vi "LIA with AM10.vi"() -> ()   [LabVIEW 2013]
uses:
  <vilib>/express/express analysis/Spectral/Block/exnSpectralBlock spectral measurements power poly.vi
  <vilib>/express/express analysis/Spectral/Block/exnSpectralBlock spectral measurements power WFM.vi
  <vilib>/express/express analysis/Spectral/XNode/ExpressSpectralMeasurementsBlockNode.xnode
panel:
  out "XY output":dbl[][](graph)=[[7.160796582041422e-23, 0.8613310626146382, 2.4561359846943875, 2.952874741807238, 1.7810719719127623, 0.28647450836648075, 0.1855399799266717, 1.5941857793632301, 2.8946647286877365, 2.5934529411128726, 1.0364745084779694, 0.011827948025126142, 0.696259807484987, 2.3037401923711305, 2.9881720520319566, 1.9635254917181835, 0.406547058891952, 0.1053352711626314, 1.405814220670607, 2.8144600200045553, 2.7135254917289764, 1.2189280280935204, 0.047125258287880584, 0.5438640153388544, 2.138668937250768, 2.999999999813988, 2.138668937326914, 0.5438640153438781, 0.04712525829527701, 1.2189280280673727, 2.7135254915392104, 2.8144600200446352, 1.405814220676119, 0.10533527116920109, 0.4065470588630961, 1.96352549160863, 2.9881720520128687, 2.3037401926017003, 0.6962598075630243, 0.011827948035904793, 1.0364745085201217, 2.593452941203313, 2.8946647287738734, 1.594185779237936, 0.18553997990325743, 0.2864745084519614, 1.7810719718442396, 2.9528747414006133, 2.4561359846600666, 0.861331062670481, 3.3077676520313965e-24, 0.8613310627550416, 2.4561359846139497, 2.9528747415820673, 1.7810719718610435, 0.28647450845342576, 0.18553997990881135, 1.5941857791936822, 2.8946647285307203, 2.5934529411452028, 1.0364745085708484, 0.01182794802446571, 0.6962598076358434, 2.3037401924693217, 2.9881720519815427, 1.9635254914432874, 0.4065470589446706, 0.10533527118504565, 1.4058142206375985, 2.814460020130084, 2.7135254916593086, 1.2189280280503507, 0.04712525828537252, 0.5438640154419273, 2.1386689373343555, 3.0000000000990474, 2.1386689374412686, 0.5438640154158645, 0.04712525831168253, 1.2189280280960597, 2.7135254916498694, 2.814460020186744, 1.4058142207416613, 0.10533527116967795, 0.40654705886722364, 1.963525491642289, 2.988172052072964, 2.3037401923713547, 0.6962598075051848, 0.011827948028521627, 1.036474508509565, 2.593452941035456, 2.894664728876174, 1.5941857792833374, 0.18553997989479157, 0.28647450845309624, 1.7810719719307495, 2.9528747417073142, 2.456135984617047, 0.8613310626750714], [6.397055649297223e-11, 1.3572405786433024, 1.1557698641977745, -0.3730348307598141, -1.4734308761192492, -0.8816778782179262, 0.7226305111206902, 1.4970400927124303, 0.5521868290009423, -1.0268206588885556, -1.4265847744961446, -0.1879998502992948, 1.266491888166919, 1.266491888200227, -0.18799985034798364, -1.4265847745588331, -1.0268206589514395, 0.5521868289985771, 1.4970400926044023, 0.7226305111386365, -0.8816778784900925, -1.4734308760566728, -0.3730348305927203, 1.155769864081423, 1.3572405786439674, 2.6015694700992775e-12, -1.3572405786883703, -1.1557698640905518, 0.37303483065207627, 1.473430876027617, 0.8816778784332103, -0.7226305111440005, -1.497040092612899, -0.5521868290321227, 1.0268206588799003, 1.426584774477441, 0.18799985035196828, -1.2664918883228173, -1.2664918883125516, 0.18799985047137116, 1.4265847745564424, 1.0268206589180475, -0.5521868290123274, -1.4970400925916614, -0.7226305110339414, 0.881677878482172, 1.473430876065951, 0.37303483070812155, -1.1557698641772307, -1.3572405787292774, 7.286958480330694e-12, 1.357240578861082, 1.1557698641619196, -0.3730348307293721, -1.473430876074467, -0.8816778784889762, 0.722630511058582, 1.497040092549754, 0.5521868289675292, -1.0268206588939026, -1.4265847746274427, -0.18799985028680116, 1.266491888443322, 1.2664918882562046, -0.18799985034827246, -1.4265847743516558, -1.0268206590880522, 0.552186829118073, 1.4970400925712481, 0.7226305111728633, -0.8816778784709165, -1.473430876002493, -0.3730348305763276, 1.1557698642970033, 1.3572405786935529, -8.590198202405667e-13, -1.3572405787589454, -1.1557698642469916, 0.3730348307839356, 1.4734308760588328, 0.8816778784711621, -0.7226305111839482, -1.4970400926806984, -0.5521868290380831, 1.0268206588923217, 1.426584774503892, 0.1879998503577455, -1.2664918881996443, -1.2664918881998886, 0.18799985035055852, 1.4265847745384521, 1.0268206588590414, -0.5521868290353029, -1.4970400926322998, -0.7226305109989726, 0.8816778784876612, 1.4734308761340573, 0.37303483075432026, -1.1557698641604481, -1.3572405787345143]] caption="Input Signal"
  out "Lock-in Output":cluster{"Ch 1 Output":dbl, "Ch 2 Output":dbl}(graph)={"Ch 1 Output"=2.99999147666684, "Ch 2 Output"=4.749187889468861e-12} caption="Lock-in Analysis"
  in  "Phase (°)":dbl caption="LOCK-IN Phase" format="%.2f"
  in  "Monitor":u16(ring) items=["Input Signal", "After Mixer"]
  out "Power Spectral Density":cluster{"f0":dbl, "df":dbl, "magnitude":dbl[]}(graph)={"f0"=0.0, "df"=0.01, "magnitude"=[-235.21607825145085, -218.3937535918811, -211.57980464454627, -219.0173516225138, -216.7688290117615, -227.34685181005236, -218.16724192412624, -214.6758364793697, -214.71830862190149, 9.542425094407328, -217.7051009330383, -220.7691633252297, -212.60929639110955, -213.01249803295275, -216.67836056343054, -214.9995950002794, -220.6607411225575, -212.65395812587005, -224.25144059753904, -218.23736966151543, -219.96657196923883, -222.76781056167866, -212.8404028730375, -214.7157786100669, -210.0824382535258, -215.8244598071573, -209.1926052730962, -211.51409381734052, -221.9697489273974, -215.1870579937338, -211.0080371535637, -230.61801872432034, -222.61555635556283, -215.12031239654422, -226.3222143787744, -213.08361230290757, -213.73344693439827, -212.09149744828164, -237.98927548601935, -221.72257852706096, -216.38992841637275, -214.7673342129894, -215.80884880067177, -207.499972356578, -215.86127934217419, -219.33399937224, -219.58911586802202, -216.03742266424695, -215.02006922582063, -218.03690366453156]}
  out "Phasor Representation of Lock-In Output":cluster{"Ch 1 Output":dbl, "Ch 2 Output":dbl}[](graph)=[{"Ch 1 Output"=2.99662702723827, "Ch 2 Output"=-2.5790815749905384e-12}, {"Ch 1 Output"=2.995358935904702, "Ch 2 Output"=-1.600659266616595e-12}, {"Ch 1 Output"=2.9945927518921893, "Ch 2 Output"=-1.1586173268220065e-12}, {"Ch 1 Output"=2.994229007813994, "Ch 2 Output"=-1.0891180515438528e-12}, {"Ch 1 Output"=2.994178400041988, "Ch 2 Output"=-7.018571078375837e-13}, {"Ch 1 Output"=2.9943625860211864, "Ch 2 Output"=1.2387460212332801e-13}, {"Ch 1 Output"=2.9947143595459833, "Ch 2 Output"=9.988247092988941e-13}, {"Ch 1 Output"=2.9951773567757507, "Ch 2 Output"=1.6429471635901913e-12}, {"Ch 1 Output"=2.9957054244850045, "Ch 2 Output"=2.3074000163604176e-12}, {"Ch 1 Output"=2.9962617612040914, "Ch 2 Output"=3.132801941572091e-12}, {"Ch 1 Output"=2.9968179221936446, "Ch 2 Output"=3.8173071586339545e-12}, {"Ch 1 Output"=2.9973527610714332, "Ch 2 Output"=3.922307228194296e-12}, {"Ch 1 Output"=2.9978513646575764, "Ch 2 Output"=3.2926514915426665e-12}, {"Ch 1 Output"=2.998304023363372, "Ch 2 Output"=2.5213873287780478e-12}, {"Ch 1 Output"=2.9987052672430683, "Ch 2 Output"=2.095662338336086e-12}, {"Ch 1 Output"=2.9990529876049297, "Ch 2 Output"=1.7451639948826307e-12}, {"Ch 1 Output"=2.9993476557183225, "Ch 2 Output"=1.0766983637301205e-12}, {"Ch 1 Output"=2.9995916434977667, "Ch 2 Output"=-7.7713426602266e-14}, {"Ch 1 Output"=2.9997886459053773, "Ch 2 Output"=-1.4843901385551484e-12}, {"Ch 1 Output"=2.9999432010043945, "Ch 2 Output"=-2.805711784224486e-12}, {"Ch 1 Output"=3.000060300921067, "Ch 2 Output"=-4.182689754747923e-12}, {"Ch 1 Output"=3.0001450852334033, "Ch 2 Output"=-5.7840254493691e-12}, {"Ch 1 Output"=3.000202607338317, "Ch 2 Output"=-7.433486148990116e-12}, {"Ch 1 Output"=3.0002376639933472, "Ch 2 Output"=-8.674989772490261e-12}, {"Ch 1 Output"=3.000254678334139, "Ch 2 Output"=-9.056488928793801e-12}, {"Ch 1 Output"=3.000257627115586, "Ch 2 Output"=-8.692276282347365e-12}, {"Ch 1 Output"=3.000250003613007, "Ch 2 Output"=-8.104261962935539e-12}, {"Ch 1 Output"=3.0002348084548918, "Ch 2 Output"=-7.494134437440875e-12}, {"Ch 1 Output"=3.0002145615773665, "Ch 2 Output"=-6.9560421124757496e-12}, {"Ch 1 Output"=3.00019132943091, "Ch 2 Output"=-6.736480378543125e-12}, {"Ch 1 Output"=3.0001667624899815, "Ch 2 Output"=-6.884063964721238e-12}, {"Ch 1 Output"=3.000142138997351, "Ch 2 Output"=-7.347238916487514e-12}, {"Ch 1 Output"=3.000118411679514, "Ch 2 Output"=-8.014782704962025e-12}, {"Ch 1 Output"=3.0000962548898635, "Ch 2 Output"=-8.601127070451612e-12}, {"Ch 1 Output"=3.0000761102732425, "Ch 2 Output"=-8.847007531240794e-12}, {"Ch 1 Output"=3.000058229590788, "Ch 2 Output"=-8.936320334688542e-12}, {"Ch 1 Output"=3.000042713802999, "Ch 2 Output"=-8.927590533950898e-12}, {"Ch 1 Output"=3.000029547880391, "Ch 2 Output"=-8.239303128363778e-12}, {"Ch 1 Output"=3.0000186311090906, "Ch 2 Output"=-6.696268700027832e-12}, {"Ch 1 Output"=3.0000098028931537, "Ch 2 Output"=-4.771497592300238e-12}, {"Ch 1 Output"=3.0000028642245966, "Ch 2 Output"=-2.808072656482772e-12}, {"Ch 1 Output"=2.9999975951124305, "Ch 2 Output"=-8.15920048923648e-13}, {"Ch 1 Output"=2.9999937683435385, "Ch 2 Output"=1.160281416825983e-12}, {"Ch 1 Output"=2.9999911599920828, "Ch 2 Output"=2.5866747361203684e-12}, {"Ch 1 Output"=2.9999895571091137, "Ch 2 Output"=3.0453247859602903e-12}, {"Ch 1 Output"=2.999988763022408, "Ch 2 Output"=2.99657373707623e-12}, {"Ch 1 Output"=2.999988600658461, "Ch 2 Output"=3.25905893169565e-12}, {"Ch 1 Output"=2.999988914265522, "Ch 2 Output"=4.051312205799775e-12}, {"Ch 1 Output"=2.999989569881677, "Ch 2 Output"=4.7268767433370936e-12}, {"Ch 1 Output"=2.9999904548535827, "Ch 2 Output"=4.886296431704625e-12}] caption="XY Graph"
  out "Time-Domain":dbl[][](graph)=[[5.7264905182118526e-11, 1.6074803850291068, 2.714481157375272, 2.976344103913628, 2.311539728422606, 0.9270509830904567, -0.7460696614724398, -2.1869058822716396, -2.9468617524061633, -2.789329457711673, -1.7633557568847291, -0.18837155849797071, 1.445261022346591, 2.628920040335509, 2.994080185279943, 2.427050983244081, 1.1043736580146353, -0.5621439439077028, -2.053641317613207, -2.905749483311644, -2.853169548811224, -1.912271969373071, -0.37599970068327676, 1.277337874669322, 2.5329837765284298, 2.999999999929249, 2.532983776596802, 1.2773378747838027, -0.3759997008364309, -1.9122719691652454, -2.85316954893021, -2.9057494834195046, -2.053641317725618, -0.5621439439232003, 1.1043736580337347, 2.427050983043902, 2.994080185337669, 2.6289200401578983, 1.4452610221701134, -0.1883715586287009, -1.7633557568382405, -2.789329457700561, -2.946861752358229, -2.1869058821346656, -0.7460696615691468, 0.9270509830480291, 2.3115397283942496, 2.9763441039140974, 2.714481157331208, 1.6074803848424404, 3.1941014126547703e-12, -1.607480384929976, -2.7144811573655114, -2.9763441038477843, -2.31153972845064, -0.9270509831065624, 0.7460696613477636, 2.1869058823191936, 2.946861752084573, 2.7893294576862684, 1.7633557570309557, 0.1883715587352395, -1.445261022233788, -2.6289200402198905, -2.99408018525837, -2.4270509830062603, -1.1043736580309171, 0.5621439437525994, 2.0536413177121613, 2.905749483546511, 2.853169548964771, 1.9122719691992385, 0.3759997007175391, -1.2773378745019865, -2.532983776459921, -3.000000000086837, -2.5329837766539796, -1.2773378745456503, 0.3759997006264955, 1.9122719691101928, 2.8531695489636224, 2.905749483361673, 2.0536413177483404, 0.5621439437392151, -1.1043736580438444, -2.427050983158539, -2.9940801853415446, -2.628920040177921, -1.4452610222029727, 0.18837155865800395, 1.7633557568570961, 2.7893294575180625, 2.9468617522226395, 2.1869058821760277, 0.7460696614997623, -0.9270509831169068, -2.3115397282190187, -2.976344103874128, -2.714481157489229, -1.6074803848518553], [-2.17504699296209e-13, 0.5358267949785253, 0.9048270524664113, 0.9921147013144053, 0.7705132427756372, 0.3090169943750446, -0.24868988716530674, -0.7289686274214977, -0.9822872507286484, -0.9297764858881211, -0.5877852522924625, -0.06279051952964025, 0.48175367410192665, 0.8763066800438156, 0.9980267284282992, 0.8090169943748718, 0.3681245526848752, -0.18738131458518154, -0.6845471059293632, -0.9685831611287765, -0.9510565162950781, -0.6374239897487644, -0.12533323356383602, 0.4257792915651914, 0.8443279255019028, 1.0, 0.8443279255020052, 0.4257792915653642, -0.12533323356454887, -0.6374239897486171, -0.9510565162950192, -0.9685831611285978, -0.6845471059288395, -0.1873813145862625, 0.3681245526855433, 0.8090169943752942, 0.9980267284282872, 0.8763066800439077, 0.48175367410129705, -0.06279051952944965, -0.5877852522923079, -0.9297764858883856, -0.9822872507286842, -0.7289686274216284, -0.2486898871646108, 0.30901699437486296, 0.7705132427755155, 0.9921147013144953, 0.9048270524661053, 0.5358267949794544, -9.360250641947212e-13, -0.5358267949794993, -0.9048270524661279, -0.9921147013144886, -0.7705132427754816, -0.3090169943748125, 0.2486898871646622, 0.7289686274216648, 0.9822872507286942, 0.929776485888366, 0.587785252292265, 0.0627905195293967, -0.4817536741013435, -0.8763066800439332, -0.9980267284282839, -0.809016994375263, -0.368124552685494, 0.18738131458631463, 0.6845471059288781, 0.968583161128611, 0.9510565162950028, 0.6374239897485763, 0.12533323356449624, -0.42577929156541217, -0.8443279255020336, -1.0, -0.8443279255018744, -0.4257792915651434, 0.12533323356388867, 0.6374239897488052, 0.9510565162950946, 0.9685831611287633, 0.6845471059293246, 0.1873813145851294, -0.36812455268492456, -0.809016994374903, -0.9980267284283025, -0.8763066800437901, -0.4817536741018802, 0.06279051952969321, 0.5877852522925053, 0.9297764858881407, 0.9822872507286384, 0.7289686274214614, 0.24868988716525536, -0.30901699437509506, -0.770513242775671, -0.9921147013144119, -0.9048270524663886, -0.5358267949784805]] caption="Input Signal"
  in  "Tab Control":enum32{"Main Settings ", "Other Settings"}(tab)
  in  "Sinusoidal\nInput\nSettings":cluster{"fc (Hz)":dbl, "Ac (V)":dbl}[](array[cluster])=[{"fc (Hz)"=60.0, "Ac (V)"=1.0}]
  out "CH Y Output (V)":dbl(knob)=4.749187889468861e-12 caption="CH 2 Output" scale=-5.0..5.0
  out "CH X Output (V)":dbl(knob)=2.99999147666684 caption="CH 1 Output" scale=-5.0..5.0
  in  "Frequency fS (Hz)":dbl=90.0 caption="Frequency" format="%.2f"
  in  "Amplitude AS (V)":dbl=3.0 caption="Amplitude" format="%.2f"
  in  "AM Percentage (%)":dbl caption="Noise Amplitude" min=0.0 max=100.0
  in  "Phase  f (°)":dbl caption="Phase Angle" format="%.2f"
  in  "AM Freq fAM (Hz)":dbl=1.0 caption="Noise Amplitude" format="%.4f"
  in  "Auto-Track":bool=TRUE caption="Auto-Tracking"
  in  "Low-Pass Filter":bool=TRUE
  in  "Time Constant t (s)":dbl=3.0 caption="Time Constant (sec)" format="%#.1p"
  in  "Rolloff":sgl(ring)=2.0 caption="Low-pass filter slope" items=["None", "6 dB/oct", "12 dB/oct", "18 dB/oct", "24 dB/oct"]
  in  "Ref  Freq  fR (Hz)":dbl=90.0 caption="Manual Set" format="%.2f"
  in  "(V)":dbl=1e-11 caption="Noise Amplitude" min=1e-11 format="%.4f"
  in  "Enable sinusoidal inputs":bool
  out "Ch 1 Output":dbl=2.99999147666684 format="%.2f"
  out "Ch 2 Output":dbl=4.749187889468861e-12 format="%.2f"
  out "Magnitude":dbl=2.99999147666684 caption="Input Signal Amp" format="%.2f"
  out "Phase":dbl=9.070306509121702e-11 caption="Phase Difference" format="%.2f"
  out "Sampling Freq.":dbl=1000.0 format="%.2f"
  in  "IntegrationPeriod(s)":dbl=0.1 format="%#_6p"
  in  "Sampling Int. (s)":dbl=0.001 caption="Sampling Int. (ms)" format="%.3f"
  # ","
  # "Input Signal"
  # "Lockin Output"
  # "Lockin Settings"
  # "Additional Signals"
  # "noise"
  # "Lock-In Output"
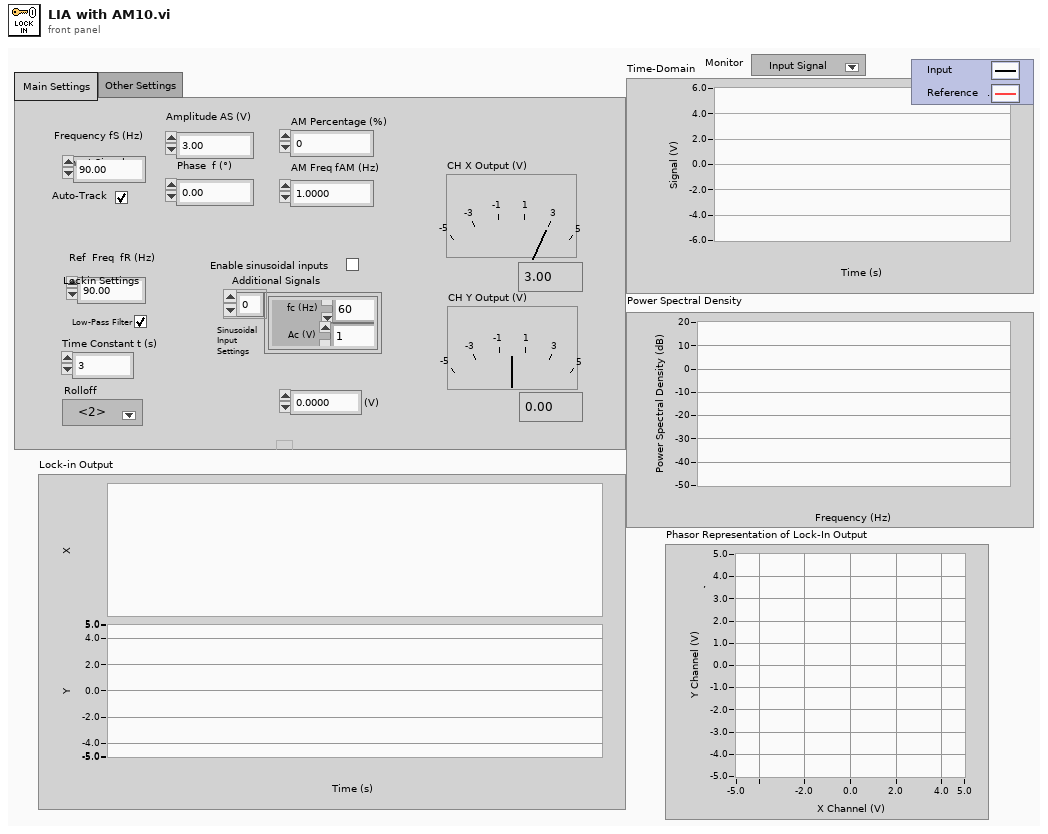
[diagram p1: front panel]
types:
  T1 = cluster{"averaging mode":u16, "weighting mode":u16, "number of averages":u32}
  T2 = cluster{"dB On (F)":bool, "unwrap phase (F)":bool, "convert to degree (F)":bool}
  T3 = cluster{"Amplitude AS (V)":dbl, " Frequency fS (Hz)":dbl, "Phase  f (°)":dbl, dbl, "Rolloff":sgl, "Time Constant t (s)":dbl, bool, " Phase (°)":dbl, " Frequency fS (Hz)":dbl, dbl, "AM Freq fAM (Hz)":dbl, "Sampling Int. (s)":dbl, dbl}
  T4 = cluster{"Amplitude":dbl, "Frequency":dbl, "Phase Angle":dbl, "Spectral Amplitude":dbl, "Time":dbl, "Low-pass filter scope":dbl, "Time Constant (sec)":dbl, "Reset Filters":bool, "LOCK-IN Phase":dbl, "LOCK-IN Freq":dbl, "Sampling-Int(ms)":dbl, "Reference Signal":cluster{dbl[], dbl[]}, "Input Signal":dbl[], "N":i32}
  T5 = cluster{"Amplitude":dbl, "Frequency":dbl, "Phase Angle":dbl, "Noise Amplitude":dbl, "Time":dbl, "Low-pass filter slope":dbl, "Time Constant (sec)":dbl, "Reset Filters":bool, "LOCK-IN Phase":dbl, "LOCK-IN Freq":dbl, "Input Signal":dbl[], "Ch 1 Mult":dbl, "Ch 2 Mult":dbl, "Reference Signal":cluster{dbl[], dbl[]}}
  T6 = cluster{"Ch 1 Output":dbl, "Ch 2 Output":dbl, "Input Signal Amp":dbl, "Phase Difference":dbl, "X-Y Data":cluster{"Current Queue":dbl[], "Current Queue":dbl[]}, "Input Signal":dbl[], "Reference Signal":cluster{dbl[], dbl[]}}
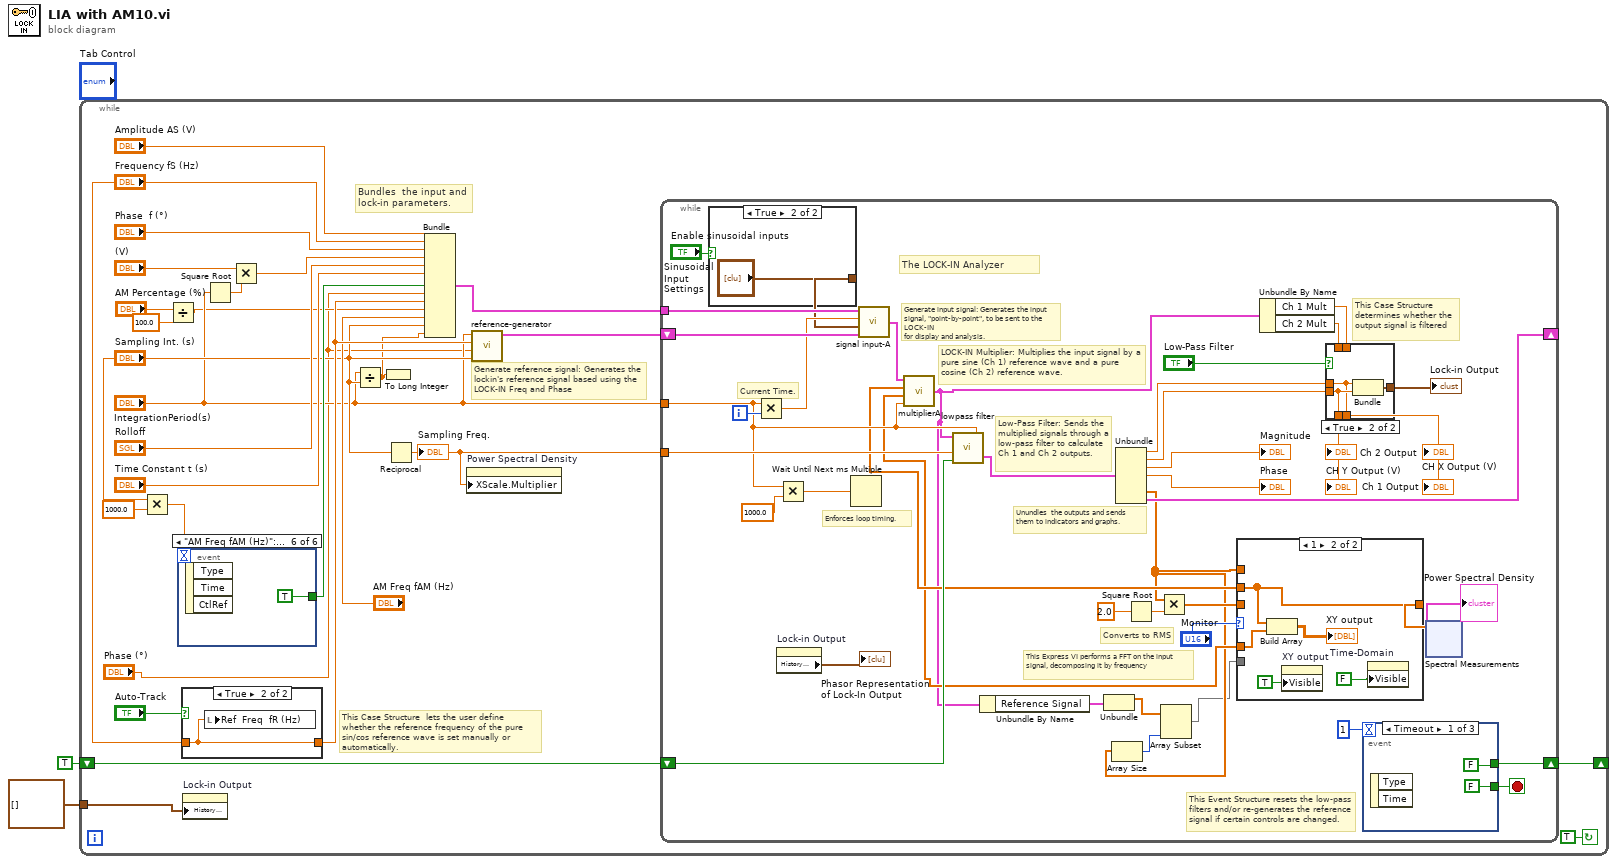
[diagram p0: block diagram]
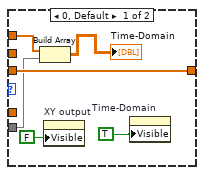
[diagram p2: hidden frame]
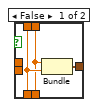
[diagram p3: hidden frame]
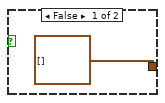
[diagram p4: hidden frame]
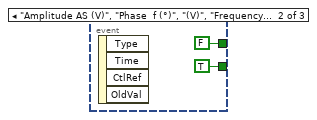
[diagram p5: hidden frame]
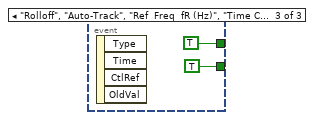
[diagram p6: hidden frame]
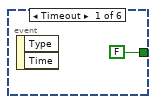
[diagram p7: hidden frame]
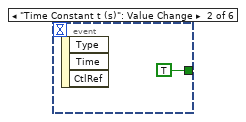
[diagram p8: hidden frame]
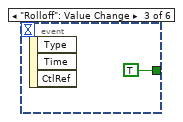
[diagram p9: hidden frame]
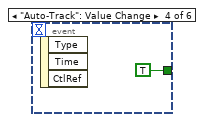
[diagram p10: hidden frame]
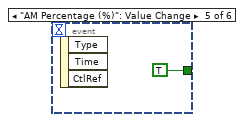
[diagram p11: hidden frame]
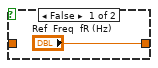
[diagram p12: hidden frame]
diagram:
  n1 = while {
    shift-right: [w22] -> _
    shift-left: TRUE -> [w23]
    tunnel: cluster{"Ch 1 Output":dbl, "Ch 2 Output":dbl}[] [] ("History Data") -> [w4]
    stop <- TRUE continue-if-true
    # "Generate reference signal: Generates the \nlockin's reference signal based using the \nLOCK-IN Freq and Phase"
    # "This Case Structure  lets the user define whether the reference frequency of the pure sin/cos reference wave is set manually or automatically."
    # "Bundles  the input and lock-in parameters."
    n2 = Multiply(x="Sampling Int. (s)", y=1000.0) -> (x*y=w16:dbl)
    n3 = Divide(x="AM Percentage (%)", y=100.0) -> (x/y=w6:dbl)
    n4 = event shown="[5] \"AM Freq fAM (Hz)\": Value Change" {
      selector: _ -> [_ _ _ _ _ _]
      dyn-events: _ -> [_ _ _ _ _ _]
      timeout: w16 -> [_ _ _ _ _ _]
      tunnel: [FALSE TRUE TRUE TRUE TRUE TRUE] -> w19
      event Timeout {
        n5 = event-data() -> ()  [unwired: 1 in, 2 out]
      }
      event "Time Constant t (s)": Value Change {
        n6 = event-data() -> ()  [unwired: 1 in, 3 out]
      }
      event "Rolloff": Value Change {
        n7 = event-data() -> ()  [unwired: 1 in, 3 out]
      }
      event "Auto-Track": Value Change {
        n8 = event-data() -> ()  [unwired: 1 in, 3 out]
      }
      event "AM Percentage (%)": Value Change {
        n9 = event-data() -> ()  [unwired: 1 in, 3 out]
      }
      event "AM Freq fAM (Hz)": Value Change {
        n10 = event-data() -> ()  [unwired: 1 in, 3 out]
      }
    }
    n11 = case shown="True" "Auto-Track" {
      tunnel: ["Ref  Freq  fR (Hz)" w114] -> w18
      tunnel: "Frequency fS (Hz)" -> [_ w114]
      frame False {
      }
      frame True {
        n12 = local write "Ref  Freq  fR (Hz)"(w114) -> ()
      }
    }
    n13 = property on="Lock-in Output" class="WFChart (strict)"("History Data"=w4) -> ()  [unwired: 2 in, 2 out]
    n14 = Square Root(x="IntegrationPeriod(s)") -> (sqrt(x)=w10:dbl)
    n15 = Multiply(x="(V)", y=w10) -> (x*y=w11:dbl)
    n16 = Divide(x="IntegrationPeriod(s)", y="Sampling Int. (s)") -> (x/y=w3:dbl)
    n17 = To Long Integer(number=w3) -> ()  [unwired: 1 out]
    n18 = Reciprocal(x="Sampling Int. (s)") -> (1/x=w24:dbl)
    "Sampling Freq." <- w24
    n19 = Bundle("Amplitude AS (V)"="Amplitude AS (V)", "Frequency fS (Hz)"="Frequency fS (Hz)", "Phase  f (°)"="Phase  f (°)", w11, "Rolloff"="Rolloff", "Time Constant t (s)"="Time Constant t (s)", w19, "Phase (°)"="Phase (°)", "Frequency fS (Hz)"=w18, w6, "AM Freq fAM (Hz)"="AM Freq fAM (Hz)", "Sampling Int. (s)"="Sampling Int. (s)", w3) -> (w26:T3)  [unwired: 1 in]
    n20 = property on="Power Spectral Density" class="WFGraph (strict)"("XScale.Multiplier"=w24) -> ()  [unwired: 2 in, 2 out]
    n21 = call "reference-generator.vi"("SamplingInt(s)"="Sampling Int. (s)", "LockinPhase"="Phase (°)", "LockinFreq"=w18, "IntegrationPeriod(s)"="IntegrationPeriod(s)") -> ("output cluster"=w25:cluster{dbl[], dbl[]})  [unwired: 7 in]
    n22 = while {
      tunnel: w24 -> [w61]
      tunnel: w26 -> [w67]
      tunnel: "IntegrationPeriod(s)" -> [w49]
      shift-right: [w68] -> _
      shift-left: w25 -> [w66]
      shift-right: [w58] -> w22
      shift-left: w23 -> [w59]
      i -> [w64]
      stop <- w60 stop-if-true
      # "This Case Structure  determines whether the output signal is filtered"
      # "Converts to RMS"
      # "This Express VI performs a FFT on the input signal, decomposing it by frequency"
      # "Enforces loop timing."
      # "Current Time."
      # "This Event Structure resets the low-pass filters and/or re-generates the reference signal if certain controls are changed."
      # "The LOCK-IN Analyzer"
      # "Unundles  the outputs and sends them to indicators and graphs."
      # "Low-Pass Filter: Sends the multiplied signals through a low-pass filter to calculate Ch 1 and Ch 2 outputs."
      # "LOCK-IN Multiplier: Multiplies the input signal by a pure sine (Ch 1) reference wave and a pure cosine (Ch 2) reference wave."
      # "Generate input signal: Generates the input signal, \"point-by-point\", to be sent to the LOCK-IN \nfor display and analysis."
      n23 = case shown="True" "Enable sinusoidal inputs" {
        tunnel: [cluster{"F":dbl, "Ampl":dbl}[] [] ("Coherent Noise") "Sinusoidal\nInput\nSettings"] -> w51
        frame False {
        }
        frame True {
        }
      }
      n24 = Multiply(x=w49, y=w64) -> (x*y=w65:dbl)
      n25 = property on="Lock-in Output" class="WFChart (strict)"() -> ("History Data"=→"Phasor Representation of Lock-In Output":cluster{"Ch 1 Output":dbl, "Ch 2 Output":dbl}[])  [unwired: 2 in, 2 out]
      n26 = Multiply(x=w49, y=1000.0) -> (x*y=w56:dbl)
      n27 = Wait Until Next ms Multiple(millisecond multiple=w56) -> ()  [unwired: 1 out]
      n28 = call "signal input-A.vi"("Reference Signal"=w66, "Coherent Noise"=w51, "Time"=w65, "Input"=w67) -> ("OUTPUT"=w38:T4)
      n29 = call "multiplierA.vi"("Integration Period (s)"=w49, "Input"=w38) -> ("OUTPUT"=w31:T5, "ymod"=w40:dbl[], "xmod"=w41:dbl[])
      n30 = call "lowpass filter.vi"("Integration Period (s)"=w49, "initialize filters"=w59, "Sampling Freq"=w61, "INPUT"=w31) -> ("OUTPUT"=w62:T6)  [unwired: 1 in]
      n31 = Unbundle By Name(w31) -> ("Reference Signal"=w37:cluster{dbl[], dbl[]})
      n32 = Unbundle(w37) -> (w35:dbl[])  [unwired: 1 out]
      n33 = Unbundle(w62) -> ("Ch 1 Output"=w70:dbl, "Ch 2 Output"=w69:dbl, "Input Signal Amp"=→"Magnitude":dbl, "Phase Difference"=→"Phase":dbl, "Input Signal"=w34:dbl[], "Reference Signal"=w68:cluster{dbl[], dbl[]})  [unwired: 1 out]
      n34 = Array Size(array=w34) -> (size(s)=w36:i32)
      n35 = Square Root(x=2.0) -> (sqrt(x)=w55:dbl)
      n36 = Multiply(x=w34, y=w55) -> (x*y=w44:dbl[])
      n37 = Array Subset(array=w35, length=w36) -> (w33:dbl[])  [unwired: 1 in]
      n38 = case shown="1" "Monitor" {
        tunnel: w44 -> [w78 _]
        tunnel: [w78 w83] -> w43
        tunnel: w41 -> [_ w83]
        tunnel: w34 -> [w77 _]
        tunnel: w40 -> [_ w82]
        tunnel: w33 -> [w76 _]
        frame 0, Default {
          n39 = Build Array(w77, w76) -> (→"Time-Domain":dbl[][])
          n40 = property on="XY output" class="WFGraph (strict)"("Visible"=FALSE) -> ()  [unwired: 2 in, 2 out]
          n41 = property on="Time-Domain" class="WFGraph (strict)"("Visible"=TRUE) -> ()  [unwired: 2 in, 2 out]
        }
        frame 1 {
          n42 = Build Array(w83, w82) -> (→"XY output":dbl[][])
          n43 = property on="XY output" class="WFGraph (strict)"("Visible"=TRUE) -> ()  [unwired: 2 in, 2 out]
          n44 = property on="Time-Domain" class="WFGraph (strict)"("Visible"=FALSE) -> ()  [unwired: 2 in, 2 out]
        }
      }
      n45 = Unbundle By Name(w31) -> ("Ch 1 Mult"=w47:dbl, "Ch 2 Mult"=w48:dbl)
      n46 = case shown="True" "Low-Pass Filter" {
        tunnel: w70 -> [_ w87]
        tunnel: w69 -> [_ w88]
        tunnel: [w86 w89] -> w39
        tunnel: w48 -> [w85 _]
        tunnel: w47 -> [w84 _]
        tunnel: [w85 w88] -> w46
        tunnel: [w84 w87] -> w45
        frame False {
          n47 = Bundle("Ch 1 Mult"=w84, "Ch 2 Mult"=w85) -> (w86:cluster{"Ch 1 Mult":dbl, "Ch 2 Mult":dbl})  [unwired: 1 in]
        }
        frame True {
          n48 = Bundle("Ch 1 Output"=w87, "Ch 2 Output"=w88) -> (w89:cluster{"Ch 1 Output":dbl, "Ch 2 Output":dbl})  [unwired: 1 in]
        }
      }
      "Ch 1 Output" <- w45
      "Ch 2 Output" <- w46
      "CH X Output (V)" <- w45
      "CH Y Output (V)" <- w46
      "Lock-in Output" <- w39
      n49 = event shown="[0] Timeout" {
        selector: _ -> [_ _ _]
        dyn-events: _ -> [_ _ _]
        timeout: 1 -> [_ _ _]
        tunnel: [FALSE TRUE TRUE] -> w60
        tunnel: [FALSE FALSE TRUE] -> w58
        event Timeout {
          n50 = event-data() -> ()  [unwired: 1 in, 2 out]
        }
        event "Amplitude AS (V)", "Phase  f (°)", "(V)", "Frequency fS (Hz)": Value Change {
          n51 = event-data() -> ()  [unwired: 1 in, 4 out]
        }
        event "Rolloff", "Auto-Track", "Ref  Freq  fR (Hz)", "Time Constant t (s)", "IntegrationPeriod(s)", "Sampling Int. (s)", "AM Percentage (%)", "AM Freq fAM (Hz)": Value Change {
          n52 = event-data() -> ()  [unwired: 1 in, 4 out]
        }
      }
      n53 = xnode "Spectral Measurements"("Signals"=w43) -> ("Power Spectrum"=→"Power Spectral Density":cluster{"f0":dbl, "df":dbl, "magnitude":dbl[]})  [unwired: 1 in, 1 out]
    }
  }
